vi "START_HERE-Capacitance_Station_Main.vi"() -> ()   [LabVIEW 2020]
uses:
  Global 1.vi
panel:
  out "KeystateHP4275AInitSetup":string
  out "Error OUT : TSL":errorcluster
  out "Voltage Adjusted?":bool
  out "%DiffVoltage":dbl format="%_10g"
  out "VError":dbl format="%_10g"
  out "ReadCurrent":dbl format="%_10g"
  out "ReadVoltage":dbl format="%_10g"
  out "NewBiasVoltage":dbl format="%_10g"
  out "TargetBiasVoltage":dbl format="%_10g"
  out "Iteration Leak Comp":i32
  out "GLOBAL - Test Voltages Array":dbl[](array[numeric])
  out "error out Override":errorcluster
  in  "error in Override":errorcluster
  in  "Specific LCR Frequency ?":bool
  out "ArrayCluster2Arrays":cluster{"DUT (x)":dbl[], "DUT (y)":dbl[]}[](array[cluster])
  out "XY Graph":cluster{"DUT (x)":dbl[], "DUT (y)":dbl[]}[](graph)
  in  "Confirm Min&Max Voltage, Chart Method and Polarity Max Voltage?":bool
  out "Current DUT":i32
  out "Test Finishing : Error Out":errorcluster
  in  "Test Finishing : Error in":errorcluster
  out "error out : Before Test Setup Initialization":errorcluster
  out "error out : After Test Setup Initialization":errorcluster
  out "error out : After Confirm Configuration":errorcluster
  in  "Stop Short Cal":bool
  in  "Stop Open Cal":bool
  out "Frequency":string
  in  "Specific Frequency":T1(ring)=enum."1MHz"
  out "Date (DD/MM/YYYY)":string
  out "Test Type (OUTPUT)":string
  out "Test Fixture (OUTPUT)":string
  in  "Category":T2(ring)
  out "Device Type(OUTPUT)":string
  out "CapRun : error out":errorcluster
  in  "error in 2":errorcluster
  out "Captest?":bool
  out "Test Type":string
  in  "CONFIRM CONFIGURATION?":bool
  out "SHORT Compensation":string
  out "OPEN Compensation":string
  in  "After Cap run":bool
  in  "Generate Report : error in":errorcluster
  out "START PRESSED?":bool
  out "Status : CapRun":bool
  out "Max Test Voltages":dbl
  out "CapTest : Started":bool
  out "CapTest  : current time":timestamp
  out "CapTest CurrDUT : \nElapsed time (minutes)":dbl
  out "DUT   |  Elapsed Time (minutes)":dbl[][](array[numeric])
  in  "CapRun : error in":errorcluster
  out "LowCapMode?":bool
  out "Current Result at \nMax Test Voltages":dbl
  in  "CalOpen : error in":errorcluster
  out "CalShort : current time":timestamp
  out "OpenCal : current time":timestamp
  out "TestSigLevel : current time":timestamp
  in  "Calibration Short : Started":bool
  in  "Open Calibration : Started":bool
  in  "TestSigLevel : Started":bool
  in  "CalShort : error in":errorcluster
  in  "Calibration Short Failed":bool
  in  "Open Calibration Failed":bool
  out "Calibration Short : \nElapsed time (seconds)":dbl
  out "Calibration Open : \nElapsed time (seconds)":dbl
  out "Signal Level : \nElapsed time (seconds)":dbl
  out "Test Voltages (V)":dbl[](array[numeric])
  in  "Polarity for Max Voltage":u16(ring) items=["Positive", "Negative"]
  out "Temporary test data":dbl[][](array[numeric])
  out "error Mult_1":errorcluster
  out "DUT  |  Result":dbl[][](array[numeric])
  in  "DUT":i32=1
  out "Generate Report : error out":errorcluster
  in  "Open Calibration Successful":bool
  in  "Calibration Short Successful":bool
  out "4275A":refnum<visa-resource-name>
  out "3457A":refnum<visa-resource-name>
  out "Keithley 2400":refnum<visa-resource-name>
  in  "Stop":bool
  out "error Mult_0.1":errorcluster
  in  "Min Voltage":dbl
  in  "Start Test":bool
  in  "Max Voltage":dbl
  in  "Chart Voltage Generation Method":u16(ring) items=["Linear", "Crude Semi-Log (Short)", "Crude Semi-Log (Long)", "Bi-directional Crude Semi-Log (Short)", "Bi-directional Crude Semi-Log (Long)", "Manual Fill-In", "Threshold with Increment"]
  in  "Cal Open All Freq":bool
  in  "Cal Short Button":bool
  out "Multiplier":dbl format="%#_3g"
  in  "Device Types":u16(ring) items=["Diode (Rectifier & Zener)", "Transistor", "BRT", "MOSFET", "JFET", "SSOVP", "SIDAC", "Bidirectional Zener", "SCR or TRIAC", "Darlington Transistor", "MicroIntegration", "MOSFET with Gate Resistor", "IGBT", "IGBT with Gate Resistor", "Other"]
  out "Test Level Equal":bool
  in  "Stop Button":bool
  in  "OK Button":bool
  out "Current LCR Voltage":dbl format="%_6g"
  out "Test Level value":dbl
  in  "error in":errorcluster
  in  "Test Signal Level":string(combo)
  in  "Test Comments":string
  in  "Lot Date":timestamp=timestamp(3376684800 s since 1904-01-01) format="%<%x>T"
  in  "Lot Number":string
  in  "Test Fixtures":u16(ring) items=["Diode & Bipolar Capacitance Adapter Box 1, CAP 1, AXK", "Diode & Bipolar Capacitance Adapter Box 1, CAP 2, AXK", "Diode & Bipolar Capacitance Adapter Box 1, CAP 3, Anode - Cathode", "DIODE & BIPOLAR Multi-pin Capacitance fixture"]
  in  "Test System":u16(ring) items=["HP 4275A East Station", "HP 4980A South Station"]
  in  "Part Number":string
  in  "Request Number":string
  out "Report Array Header":string[](array[string])
  in  "Operator":u16(ring) items=["Dan McClurg", "Jason Rall", "Laura Vickers", "Daniel Henscheid", "Dwayne Pierce", "Hannah Morrison", "Charles Reyes", "Fadzly", "Hafiz", "Izwan", "GUEST"]
  # "CAPACITANCE TEST"
  # "FLOW :"
  # "1) Orange"
  # "2) Yellow"
  # "3) Lime"
  # "4) Light Blue"
  # "5) Purple"
  # "6) Red"
  # "RESULT : Capacitance(pF) / RG (Ohm)"
  # "Bias Parameter"
  # "NOTE : Test Signal Level is SEMI-AUTO\n------------------------------------------\nTest Signal Level = Osc Level (V) x Multiplier\n\nRule for Multiplier :\n\nIf Test Signal Level = 1 VRMS,  Multiplier = 1  ;\nElse Multiplier = 0.1\n\nOperator need to adjust Osc Level (V) MANUALLY"
  # "Current Result at Max Voltage before Retest Option"
  # "Verror = Bias - Read\n\nVerror / Bias Voltage\nmust be \nless than 0.001"
  # "Manual Override (OPTIONAL)\n-------------------------------\nSet Specific Frequency\nAFTER choosing TSL"
  # "Bias Current's range : AUTO"
  # "Bias = SourceMeter : K2400"
  # "Read = MultiMeter : HP3457A"
  # "Press 2 Times to Stop"
  # "Error Checking"
  # "LOCATION FOR THESE FILE :\n\ntemp_test_data.csv\ntemp_chart.bmp\n.xls\n\nWILL BE IN C:\\Capacitance_Project"
  # "PRODUCED BY : AFIQAH HASBULLAH ( SBN CZ ENG : 2021)"
  # "Get 4275A Keystate"
  # "This is for Resetting, from \nGlobal Variable"
  # "[] [AN] [BN] [CN] [DN] [FNN]"
  # "Frequency Step\n10 kHz - F11                     1 MHz - F17\n20(30) kHz - F12              2(3) MHz - F18\n40(50) kHz - F13              4(5) MHz - F19\n100 kHz - F14                   10 MHz - F20\n200(300) kHz - F15           *1 - F21\n400(500) kHz - F16           *2 - F22"
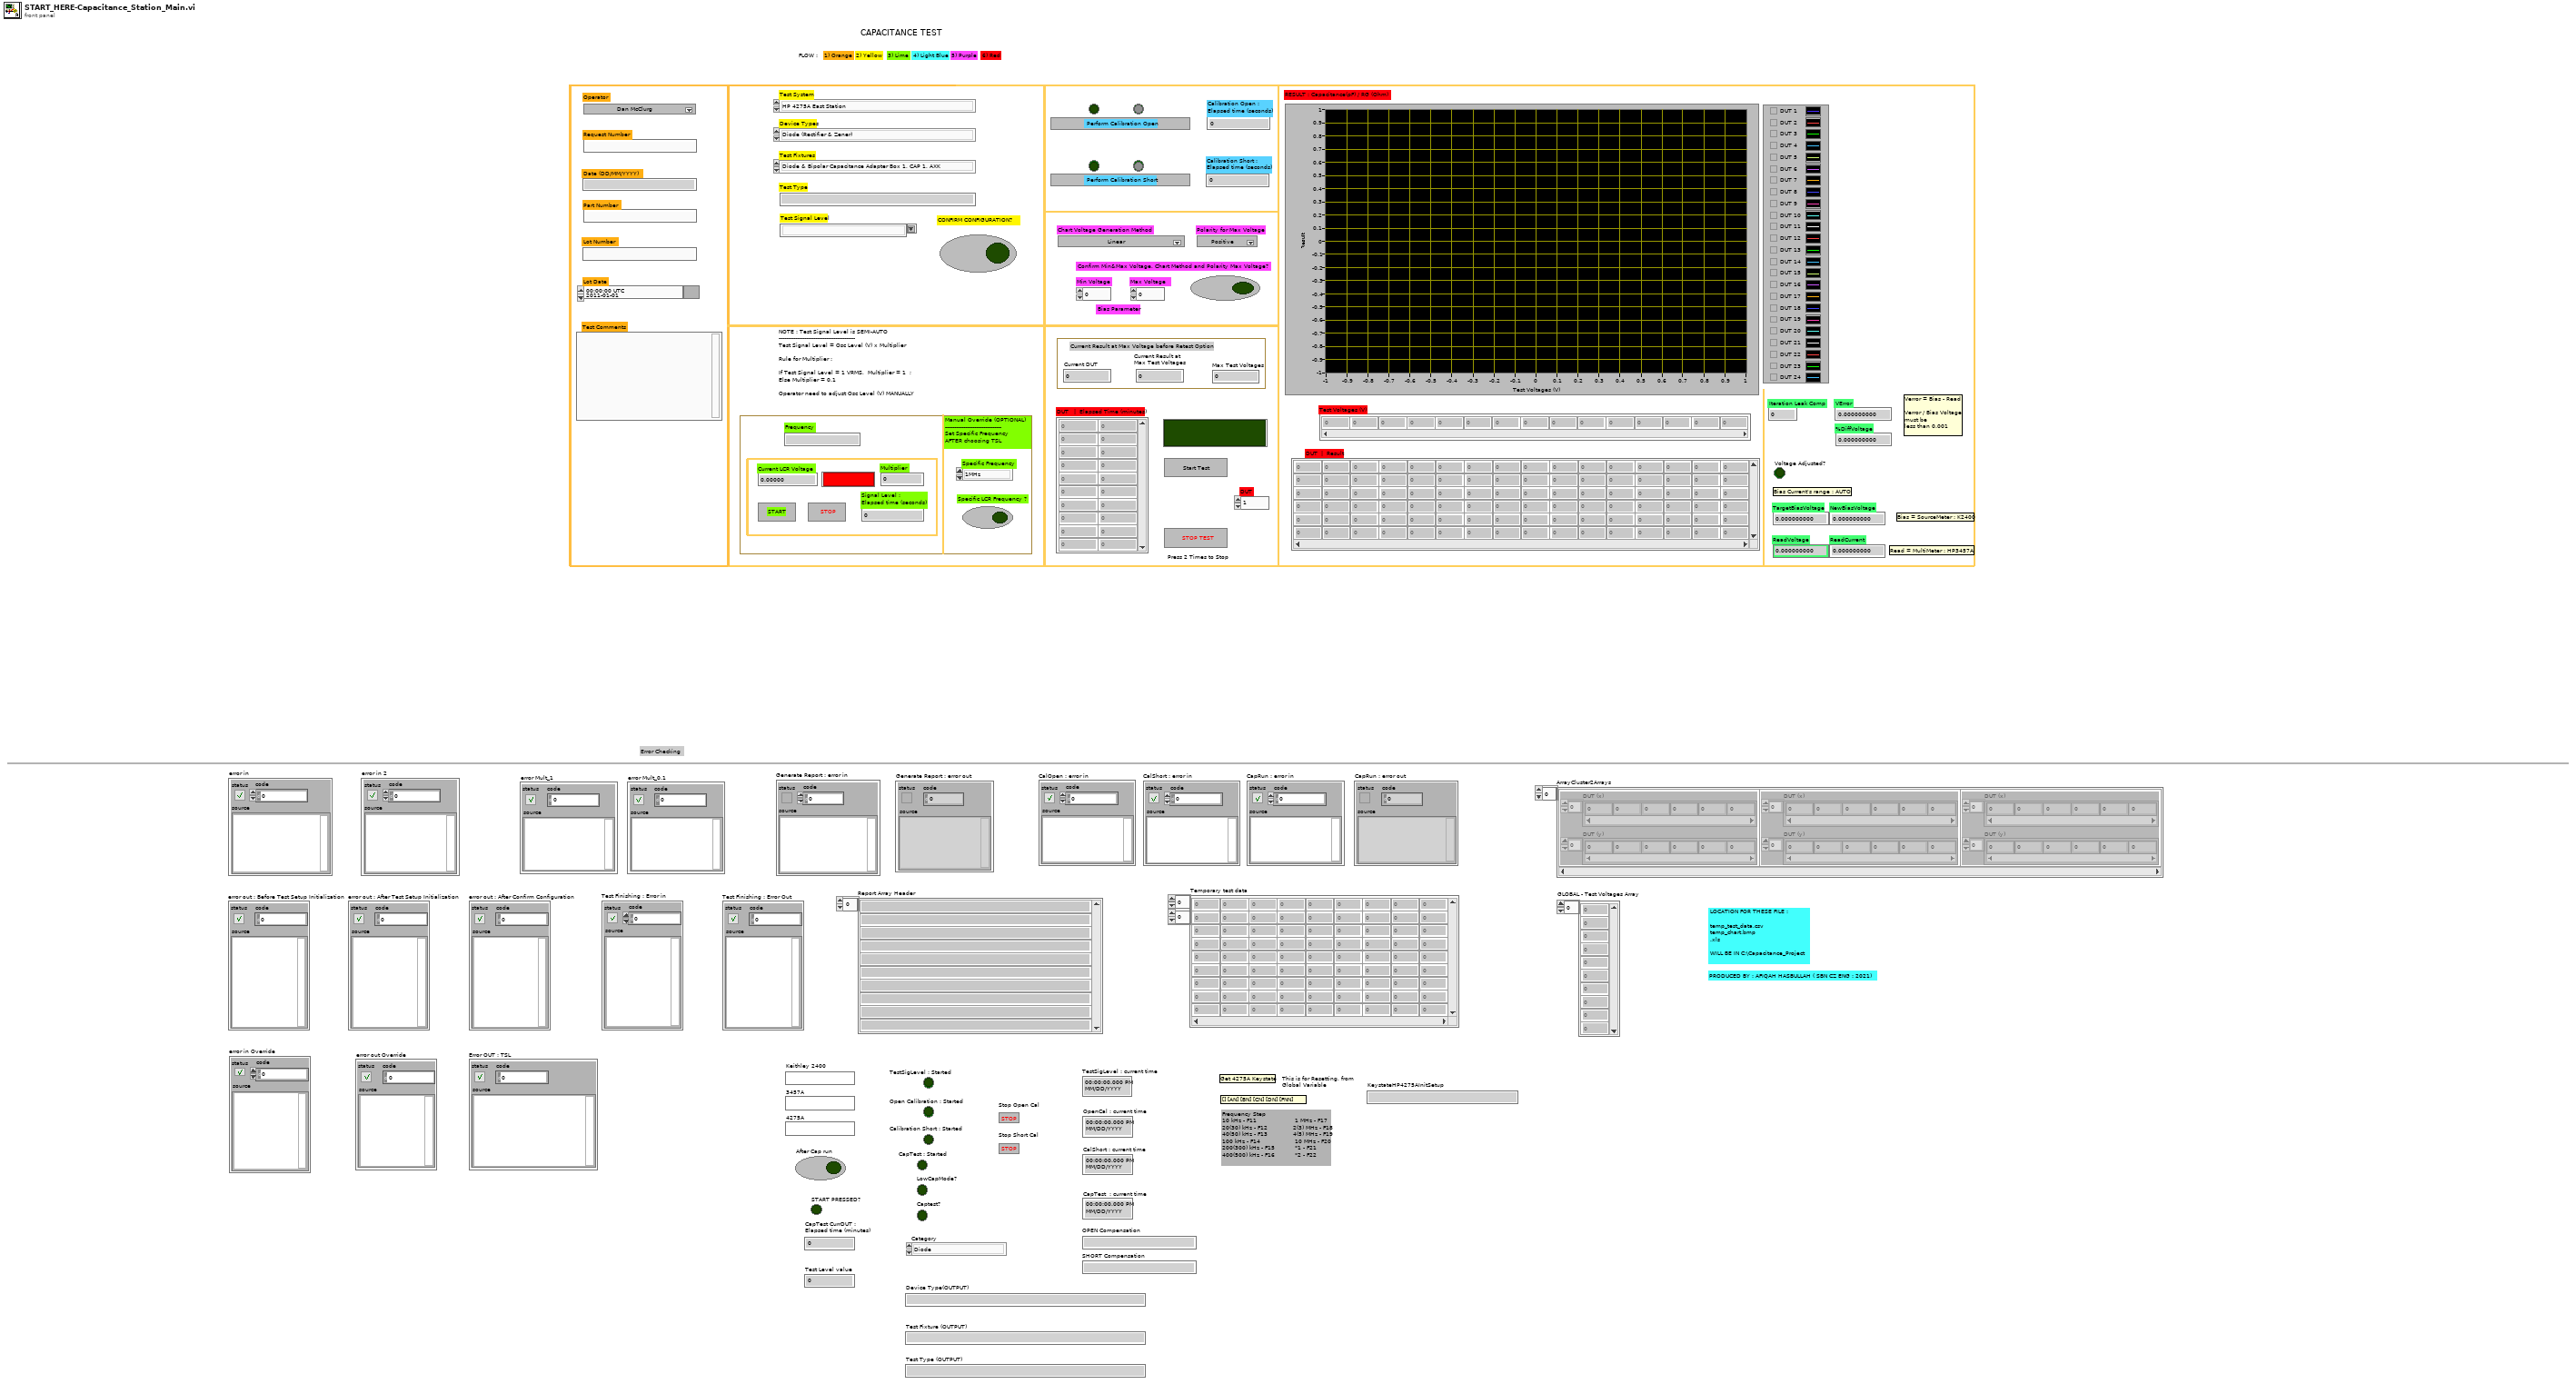
[diagram p1: front panel]
types:
  T1 = enum16{"NULL", "10kHz", "20(30)kHz", "40(50)kHz", "100kHz", "200(300)kHz", "400(500)kHz", "1MHz", "2(3)MHz", "4(5)MHz", "10MHz", "*1", "*2"}
  T2 = enum16{"Diode", "Transistor", "MOSFET", "Thyristor", "IGBT"}
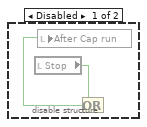
[diagram p3: hidden frame]
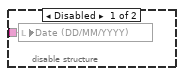
[diagram p4: hidden frame]
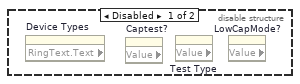
[diagram p7: hidden frame]
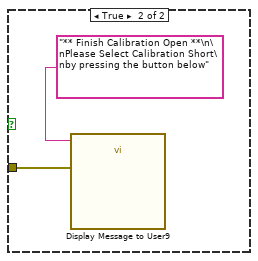
[diagram p15: hidden frame]
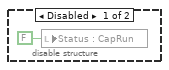
[diagram p19: hidden frame]
diagram:
  # "Manual Override"
  # "Stop Testing, Generate FULL Report"
  # "**********************************STOP **********************************"
  # "Open Calibration, Short Calibration, Start Testing"
  # "**********************************READ & WRITE **********************************"
  # "Initializing Variable"
  # "**********************************START**********************************"
  # "Test Configuration, Report Header, Test Signal Level"
  # "**********************************CONFIGURE**********************************"
  # "LOCAL VARIABLE"
  n1 = disable-structure shown="Enabled" {
    frame Enabled {
      w4 = 0.0
      w6 = 100 ("dimension size")
      w15 = 24 ("dimension size")
      w3 = "" ("Test Type (OUTPUT)")
      w17 = u16 0 items=[""]
      w5 = FALSE
      w13 = 0.0 ("Signal Level : Elapsed time (seconds)")
      w11 = 1 ("Next Part")
      w14 = 0.0 ("element")
      # "Bias Current is always in the range of 10mA"
      # "DUT 24"
      # "DUT 23"
      # "DUT 22"
      # "DUT 21"
      # "DUT 20"
      # "DUT 19"
      # "DUT 18"
      # "DUT 17"
      # "DUT 16"
      # "DUT 15"
      # "DUT 14"
      # "DUT 13"
      # "DUT 12"
      # "DUT 11"
      # "DUT 10"
      # "DUT 9"
      # "DUT 8"
      # "DUT 7"
      # "DUT 6"
      # "DUT 5"
      # "DUT 4"
      # "DUT 3"
      # "DUT 2"
      # "DUT 1"
      # "Array of cluster of Array"
      # "Must have 24 array"
      n2 = Initialize Array(w14, w6, w6) -> (w7:dbl[][])
      n3 = Initialize Array(w14) -> (w24:dbl[])  [unwired: 1 in]
      n4 = Initialize Array(w14, w15, w15) -> (w19:dbl[][])
      n5 = Initialize Array(w14, w15, 2 ("dimension size")) -> (w20:dbl[][])
      n6 = local write "Current DUT"(w11) -> ()
      n7 = local write "DUT"(w11) -> ()
      n8 = local write "Device Types"(w17) -> ()
      n9 = local write "Test Fixtures"(w17) -> ()
      n10 = local write "DUT  |  Result"(w7) -> ()
      n11 = local write "Temporary test data"(w19) -> ()
      n12 = local write "DUT   |  Elapsed Time (minutes)"(w20) -> ()
      n13 = local write "Test Voltages (V)"(w24) -> ()
      n14 = call "Device_GPIB_Addresses.vi"() -> ("HP 4275A Address"=→"4275A":refnum<visa-resource-name>, "HP 3457A Address"=→"3457A":refnum<visa-resource-name>, "Keithley 2400 Address"=→"Keithley 2400":refnum<visa-resource-name>)  [unwired: 9 in]
      n15 = local write "CapTest CurrDUT : \nElapsed time (minutes)"(w13) -> ()
      n16 = local write "Max Test Voltages"(w13) -> ()
      n17 = local write "Current Result at \nMax Test Voltages"(w13) -> ()
      n18 = local write "Signal Level : \nElapsed time (seconds)"(w13) -> ()
      n19 = local write "Calibration Open : \nElapsed time (seconds)"(w13) -> ()
      n20 = local write "Calibration Short : \nElapsed time (seconds)"(w13) -> ()
      n21 = local write "Current LCR Voltage"(w13) -> ()
      n22 = local write "Multiplier"(w13) -> ()
      n23 = local write "XY Graph"(cluster{"DUT (x)":dbl[], "DUT (y)":dbl[]}[] [{"DUT (x)"=[0.0], "DUT (y)"=[0.0]}, {"DUT (x)"=[0.0], "DUT (y)"=[0.0]}, {"DUT (x)"=[0.0], "DUT (y)"=[0.0]}, {"DUT (x)"=[0.0], "DUT (y)"=[0.0]}, {"DUT (x)"=[0.0], "DUT (y)"=[0.0]}, {"DUT (x)"=[0.0], "DUT (y)"=[0.0]}, {"DUT (x)"=[0.0], "DUT (y)"=[0.0]}, {"DUT (x)"=[0.0], "DUT (y)"=[0.0]}, {"DUT (x)"=[0.0], "DUT (y)"=[0.0]}, {"DUT (x)"=[0.0], "DUT (y)"=[0.0]}, {"DUT (x)"=[0.0], "DUT (y)"=[0.0]}, {"DUT (x)"=[0.0], "DUT (y)"=[0.0]}, {"DUT (x)"=[0.0], "DUT (y)"=[0.0]}, {"DUT (x)"=[0.0], "DUT (y)"=[0.0]}, {"DUT (x)"=[0.0], "DUT (y)"=[0.0]}, {"DUT (x)"=[0.0], "DUT (y)"=[0.0]}, {"DUT (x)"=[0.0], "DUT (y)"=[0.0]}, {"DUT (x)"=[0.0], "DUT (y)"=[0.0]}, {"DUT (x)"=[0.0], "DUT (y)"=[0.0]}, {"DUT (x)"=[0.0], "DUT (y)"=[0.0]}, {"DUT (x)"=[0.0], "DUT (y)"=[0.0]}, {"DUT (x)"=[0.0], "DUT (y)"=[0.0]}, {"DUT (x)"=[0.0], "DUT (y)"=[0.0]}, {"DUT (x)"=[0.0], "DUT (y)"=[0.0]}] ("Array of DUT Cluster")) -> ()
      n24 = disable-structure shown="Enabled" {
        frame Enabled {
          w30 = "" ("KeystateHP4275AInitSetup")
          w29 = 0 ("Array Size")
          # "Global Variable Initialization"
          n25 = Initialize Array(0.0 ("element")) -> (w33:dbl[])  [unwired: 1 in]
          n26 = global write "Global 1.vi" "KeystateHP4275AInitSetup"(w30) -> ()
          n27 = global write "Global 1.vi" "Device Type-GB"(w30) -> ()
          n28 = global write "Global 1.vi" "Test Type-GB"(w30) -> ()
          n29 = global write "Global 1.vi" "Test Comment-GB"(w30) -> ()
          n30 = global write "Global 1.vi" "Array Size"(w29) -> ()
          n31 = global write "Global 1.vi" "Iteration Leak Comp"(w29) -> ()
          n32 = global write "Global 1.vi" "DUT"(w29) -> ()
          n33 = global write "Global 1.vi" "Result - Test Voltages Array"(w33) -> ()
          n34 = global write "Global 1.vi" "~~ FINISH ~~"(FALSE ("~~ FINISH ~~")) -> ()
          n35 = global write "Global 1.vi" "error out"(errorcluster {"status"=FALSE, "code"=0, "source"=""} ("error out")) -> ()
        }
        frame Disabled {
        }
      }
      n36 = local write "%DiffVoltage"(w4) -> ()
      n37 = local write "VError"(w4) -> ()
      n38 = local write "ReadCurrent"(w4) -> ()
      n39 = local write "ReadVoltage"(w4) -> ()
      n40 = local write "NewBiasVoltage"(w4) -> ()
      n41 = local write "TargetBiasVoltage"(w4) -> ()
      n42 = global write "Global 1.vi" "%DiffVoltage"(w4) -> ()
      n43 = global write "Global 1.vi" "NewBiasVoltage"(w4) -> ()
      n44 = global write "Global 1.vi" "TargetBiasVoltage"(w4) -> ()
      n45 = global write "Global 1.vi" "ReadVoltage"(w4) -> ()
      n46 = global write "Global 1.vi" "ReadCurrent"(w4) -> ()
      n47 = global write "Global 1.vi" "VError"(w4) -> ()
      n48 = local write "KeystateHP4275AInitSetup"(w3) -> ()
      n49 = local write "Device Type(OUTPUT)"(w3) -> ()
      n50 = disable-structure shown="Enabled" {
        disable-tunnel: w3 -> [w28 _]
        frame Disabled {
          n51 = local write "Date (DD/MM/YYYY)"(w28) -> ()
        }
        frame Enabled {
        }
      }
      n52 = local write "Test Type (OUTPUT)"(w3) -> ()
      n53 = local write "Test Fixture (OUTPUT)"(w3) -> ()
      n54 = local write "Frequency"(w3) -> ()
      n55 = local write "Test Type"(w3) -> ()
      n56 = local write "OPEN Compensation"(w3) -> ()
      n57 = local write "SHORT Compensation"(w3) -> ()
      n58 = local write "Report Array Header"(string[] ["", "", "", "", "", "", "", "", "", "", "", "", "", "", ""] ("Report Array Header")) -> ()
      n59 = local write "Specific LCR Frequency ?"(w5) -> ()
      n60 = local write "Voltage Adjusted?"(w5) -> ()
      n61 = global write "Global 1.vi" "Voltage Adjusted?"(w5) -> ()
      n62 = local write "Stop Open Cal"(w5) -> ()
      n63 = local write "Stop Short Cal"(w5) -> ()
      n64 = local write "Test Level Equal"(w5) -> ()
      n65 = local write "Confirm Min&Max Voltage, Chart Method and Polarity Max Voltage?"(w5) -> ()
      n66 = local write "OK Button"(w5) -> ()
      n67 = local write "Stop Button"(w5) -> ()
      n68 = local write "After Cap run"(w5) -> ()
      n69 = local write "CapTest : Started"(w5) -> ()
      n70 = local write "LowCapMode?"(TRUE ("LowCapMode?")) -> ()
      n71 = local write "CONFIRM CONFIGURATION?"(w5) -> ()
      n72 = local write "Captest?"(TRUE ("Captest?")) -> ()
      n73 = local write "Calibration Short Successful"(w5) -> ()
      n74 = local write "Status : CapRun"(w5) -> ()
      n75 = local write "Calibration Short Failed"(w5) -> ()
      n76 = local write "Open Calibration Failed"(w5) -> ()
      n77 = local write "Cal Short Button"(w5) -> ()
      n78 = local write "Cal Open All Freq"(w5) -> ()
      n79 = local write "Open Calibration Successful"(w5) -> ()
      n80 = local write "Calibration Short : Started"(w5) -> ()
      n81 = local write "Open Calibration : Started"(w5) -> ()
      n82 = local write "TestSigLevel : Started"(w5) -> ()
      n83 = local write "Start Test"(w5) -> ()
      n84 = local write "Stop"(w5) -> ()
      n85 = local write "Specific LCR Frequency ?"(FALSE ("Specific LCR Frequency ?")) -> ()
      n86 = local write "CapTest  : current time"(timestamp(0 s since 1904-01-01) ("CapTest  : current time")) -> ()
      n87 = local write "TestSigLevel : current time"(timestamp(0 s since 1904-01-01) ("TestSigLevel : current time")) -> ()
      n88 = local write "OpenCal : current time"(timestamp(0 s since 1904-01-01) ("OpenCal : current time")) -> ()
      n89 = local write "CalShort : current time"(timestamp(0 s since 1904-01-01) ("CalShort : current time")) -> ()
      n90 = local write "Specific Frequency"(T1."1MHz" ("Specific Frequency")) -> ()
    }
    frame Disabled {
    }
  }
  n91 = disable-structure shown="Enabled" {
    frame Enabled {
      # "CALL ConfigGPIB\nCALL ConfigK2400\nCALL ResetHP3457\nCALL ConfigHP3457Norm"
      # "Captest?"
      # "Set Header"
      # "Test Type (OUTPUT)"
      # "Test Fixture (OUTPUT)"
      n92 = flat-sequence {
        tunnel: [w94] -> w54
        tunnel: [w93] -> w53
        tunnel: [w92] -> w52
        tunnel: [w91] -> w48
        tunnel: [w90] -> w45
        tunnel: [w89] -> w43
        tunnel: [w88] -> w39
        tunnel: [w101] -> w56
        tunnel: [w108] -> w55
        tunnel: w54 -> [w108]
        tunnel: [w107] -> w49
        tunnel: w48 -> [w107]
        tunnel: [w106] -> w46
        tunnel: w45 -> [w106]
        tunnel: [w105] -> w44
        tunnel: w43 -> [w105]
        tunnel: w39 -> [w102]
        tunnel: w56 -> [w118]
        tunnel: w55 -> [w117]
        tunnel: [w115] -> w50
        tunnel: w49 -> [w113]
        tunnel: [w113] -> w47
        tunnel: w46 -> [w112]
        tunnel: w44 -> [w110]
        frame #0 {
          n93 = control-ref of="Test Signal Level"() -> (w98:refnum<vi>)
          n94 = control-ref of="Device Types"() -> (w94:refnum<vi>)
          n95 = control-ref of="Test Fixtures"() -> (w97:refnum<vi>)
          n96 = control-ref of="Test Type"() -> (w89:refnum<vi>)
          n97 = control-ref of="CONFIRM CONFIGURATION?"() -> (w100:refnum<vi>)
          n98 = control-ref of="Category"() -> (w96:refnum<vi>)
          n99 = control-ref of="Captest?"() -> (w91:refnum<vi>)
          n100 = control-ref of="Device Type(OUTPUT)"() -> (w99:refnum<vi>)
          n101 = control-ref of="Test Fixture (OUTPUT)"() -> (w92:refnum<vi>)
          n102 = control-ref of="Test Type (OUTPUT)"() -> (w93:refnum<vi>)
          n103 = control-ref of="LowCapMode?"() -> (w90:refnum<vi>)
          n104 = call "Ref_Num_Test_Conf.vi"("Device Types"=w94, "Test Fixtures"=w97, "Test Signal Level"=w98, "Device Type (OUTPUT)"=w99, "Test Types"=w89, "Test Fixture (OUTPUT)"=w92, "Confirm Configuration"=w100, "Test Type (OUTPUT)"=w93, "error in"="error in 2", "Category"=w96, "LowCapMode?"=w90, "CAPACITANCE TEST?"=w91) -> ("error out"=w88:errorcluster)  [unwired: 3 in]
        }
        frame #1 {
          # "Wait until \nConfiguration Confirmed"
          n105 = call "Message_dialog.vi"("error in (no error)"=w102, "set delay"=2.0, "String"="Test Configuration will be Set Up\nPlease Wait...\n\n") -> ("error out"=w101:errorcluster)  [unwired: 8 in]
        }
        frame #2 {
          # "Test Type"
          # "LowCapMode?"
          # "Captest?"
          # "Device Types"
          # "Test Mode\nTrue : Cap"
          # "AUTO RANGING"
          # "RESOLUTION SETUP"
          # "Mode Setup"
          # "Default - C"
          # "FET Test Config"
          n106 = property class="Bool (strict)"(reference=w112) -> ("Value"=w111:bool)  [unwired: 1 in, 2 out]
          n107 = property class="Bool (strict)"(reference=w113) -> ("Value"=w114:bool)  [unwired: 1 in, 2 out]
          n108 = property class="Ring (strict)"(reference=w117) -> ("RingText.Text"=w116:string)  [unwired: 1 in, 2 out]
          n109 = global write "Global 1.vi" "Device Type-GB"(w116) -> ()
          n110 = property class="Str"(reference=w110) -> ("Value"=w109:string)  [unwired: 1 in, 2 out]
          n111 = global write "Global 1.vi" "Test Type-GB"(w109) -> ()
          n112 = call "FET_Test_Config_4275A.vi"("LowCapMode?"=w111, "error in"=w118, "Test Mode"=w114, "Device Type"=w116, "FET Test Configuration"=w109) -> ("error out"=w115:errorcluster)  [unwired: 6 in]
        }
      }
      n113 = disable-structure shown="Enabled" {
        disable-tunnel: [w122 _] -> w42
        disable-tunnel: "error in" -> [w121 _]
        frame Enabled {
          # "Test Setup Initialization"
          n114 = while {
            shift-right: [w128] -> w120
            shift-left: w121 -> [w129]
            stop <- w127 stop-if-true
            n115 = call <vilib>:"Beep.vi"("use system alert? (T)"=FALSE, "duration (msec)"=u32 3000, "frequency (Hz)"=u32 1000) -> ()  [unwired: 9 in]
            n116 = call "Display Message to User8"("error in (no error)"=w129) -> ("error out"=w128:errorcluster, "OK"=w127:bool)  [unwired: 9 in]
            n117 = Wait (ms)(milliseconds to wait=u32 200) -> ()  [unwired: 1 out]
          }
          "error out : Before Test Setup Initialization" <- w120
          n118 = call "Test_Setup_Initialization.vi"("HP 3457A Error In"=w120) -> ("HP 3457A Error Out"=w119:errorcluster)  [unwired: 10 in]
          "error out : After Test Setup Initialization" <- w119
          n119 = while {
            shift-right: [w132] -> w122
            shift-left: w119 -> [w133]
            stop <- w131 stop-if-true
            n120 = call "Display Message to User7"("error in (no error)"=w133) -> ("error out"=w132:errorcluster, "OK"=w131:bool)  [unwired: 9 in]
            n121 = Wait (ms)(milliseconds to wait=u32 200) -> ()  [unwired: 1 out]
          }
        }
        frame Disabled {
        }
      }
      n122 = disable-structure shown="Enabled" {
        frame Disabled {
          n123 = property on="Device Types" class="Ring (strict)" props=["RingText", "Text"]() -> ()  [unwired: 2 in, 3 out]
          n124 = property on="Captest?" class="Bool (strict)" props=["Value"]() -> ()  [unwired: 2 in, 3 out]
          n125 = property on="Test Type" class="Str" props=["Value"]() -> ()  [unwired: 2 in, 3 out]
          n126 = property on="LowCapMode?" class="Bool (strict)" props=["Value"]() -> ()  [unwired: 2 in, 3 out]
        }
        frame Enabled {
        }
      }
      n127 = global read "Global 1.vi" "Test Comment-GB"() -> (w51:string)
      n128 = control-ref of="Current LCR Voltage"() -> (w83:refnum<vi>)
      n129 = control-ref of="Test Level value"() -> (w84:refnum<vi>)
      n130 = control-ref of="Frequency"() -> (w57:refnum<vi>)
      n131 = control-ref of="OPEN Compensation"() -> (w81:refnum<vi>)
      n132 = control-ref of="SHORT Compensation"() -> (w82:refnum<vi>)
      n133 = control-ref of="Report Array Header"() -> (w87:refnum<vi>)
      n134 = control-ref of="Operator"() -> (w86:refnum<vi>)
      n135 = control-ref of="Request Number"() -> (w85:refnum<vi>)
      n136 = Merge Errors(w50, w42) -> (w60:errorcluster)
      n137 = control-ref of="Specific LCR Frequency ?"() -> (w36:refnum<vi>)
      n138 = control-ref of="Specific Frequency"() -> (w35:refnum<vi>)
      n139 = while {
        shift-right: [w136] -> w59
        shift-left: w60 -> [w137]
        stop <- w135 stop-if-true
        n140 = call "Display Message to User2"("error in (no error)"=w137) -> ("error out"=w136:errorcluster, "OK"=w135:bool)  [unwired: 9 in]
        n141 = Wait (ms)(milliseconds to wait=u32 200) -> ()  [unwired: 1 out]
      }
      n142 = control-ref of="Stop"() -> (w41:refnum<vi>)
      n143 = control-ref of="Date (DD/MM/YYYY)"() -> (w78:refnum<vi>)
      n144 = control-ref of="Lot Date"() -> (w77:refnum<vi>)
      n145 = call "Ref_Num_OverrideSpec.vi"("error in"="error in Override", "Specific Frequency"=w35, "Set LCR Frequency"=w36) -> ("error out"=→"error out Override":errorcluster)  [unwired: 8 in]
      n146 = control-ref of="Open Calibration : Started"() -> (w79:refnum<vi>)
      n147 = control-ref of="Calibration Short : Started"() -> (w80:refnum<vi>)
      n148 = control-ref of="Part Number"() -> (w76:refnum<vi>)
      n149 = control-ref of="Test Comments"() -> (w73:refnum<vi>)
      n150 = control-ref of="Lot Number"() -> (w74:refnum<vi>)
      n151 = control-ref of="Test System"() -> (w75:refnum<vi>)
      n152 = call "Ref_Num_Set_Header.vi"("Report Array Header"=w87, "Test Fixture (OUTPUT)"=w52, "Frequency"=w57, "Test Type (OUTPUT)"=w53, "AddTestComment"=w51, "Test Level value"=w84, "Current LCR Voltage"=w83, "Operator"=w86, "SHORT Compensation"=w82, "Request Number"=w85, "OPEN Compensation"=w81, "Date (DD/MM/YYYY)"=w78, "Calibration Short : Started"=w80, "Captest?"=w47, "Open Calibration : Started"=w79, "Lot Date"=w77, "Part Number"=w76, "Test System"=w75, "Lot Number"=w74, "Test Comments"=w73, "Stop"=w41) -> ()  [unwired: 7 in]
      n153 = control-ref of="Test Signal Level"() -> (w64:refnum<vi>)
      n154 = control-ref of="TestSigLevel : Started"() -> (w63:refnum<vi>)
      n155 = control-ref of="Multiplier"() -> (w65:refnum<vi>)
      n156 = control-ref of="OK Button"() -> (w62:refnum<vi>)
      n157 = control-ref of="Stop Button"() -> (w61:refnum<vi>)
      n158 = control-ref of="Test Level Equal"() -> (w66:refnum<vi>)
      n159 = control-ref of="Test Level value"() -> (w67:refnum<vi>)
      n160 = control-ref of="Current LCR Voltage"() -> (w68:refnum<vi>)
      n161 = control-ref of="TestSigLevel : current time"() -> (w69:refnum<vi>)
      n162 = control-ref of="Signal Level : \nElapsed time (seconds)"() -> (w70:refnum<vi>)
      n163 = call "Ref_Num_Set_VRMS.vi"("Multiplier"=w65, "Test Level Equal"=w66, "Test Level value"=w67, "Current LCR Voltage"=w68, "TestSigLevel : current time"=w69, "Test Signal Level"=w64, "Signal Level : Elapsed time (seconds)"=w70, "error IN"=w59, "TestSigLevel : Started"=w63, "OK Button"=w62, "Stop Button"=w61) -> ("Error OUT"=→"Error OUT : TSL":errorcluster, "error Mult_0.1"=→"error Mult_0.1":errorcluster, "error Mult_1"=→"error Mult_1":errorcluster)  [unwired: 2 in]
      "error out : After Confirm Configuration" <- w50
    }
    frame Disabled {
    }
  }
  n164 = disable-structure shown="Enabled" {
    frame Enabled {
      # "Capacitance Test"
      # "Needs to be looked at and verified."
      n165 = control-ref of="Stop"() -> (w146:refnum<vi>)
      n166 = control-ref of="After Cap run"() -> (w147:refnum<vi>)
      n167 = control-ref of="Start Test"() -> (w145:refnum<vi>)
      n168 = control-ref of="CapTest CurrDUT : \nElapsed time (minutes)"() -> (w142:refnum<vi>)
      n169 = control-ref of="Current DUT"() -> (w138:refnum<vi>)
      n170 = control-ref of="DUT"() -> (w143:refnum<vi>)
      n171 = control-ref of="DUT   |  Elapsed Time (minutes)"() -> (w144:refnum<vi>)
      n172 = while {
        tunnel: w147 -> [w189]
        tunnel: w146 -> [w188]
        tunnel: w145 -> [w184]
        tunnel: w144 -> [w187]
        tunnel: w143 -> [w186]
        tunnel: w142 -> [w185]
        tunnel: w138 -> [w170]
        stop <- w174 stop-if-true
        n173 = global read "Global 1.vi" "Result - Test Voltages Array"() -> (→"GLOBAL - Test Voltages Array":dbl[])
        n174 = global read "Global 1.vi" "ArrayCluster2Arrays"() -> (→"ArrayCluster2Arrays":cluster{"DUT (x)":dbl[], "DUT (y)":dbl[]}[])
        n175 = global read "Global 1.vi" "Iteration Leak Comp"() -> (→"Iteration Leak Comp":i32)
        n176 = property class="Bool (strict)"(reference=w188) -> ("Value"=w174:bool)  [unwired: 1 in, 2 out]
        n177 = Wait (ms)(milliseconds to wait=u32 200) -> ()  [unwired: 1 out]
        n178 = global read "Global 1.vi" "%DiffVoltage"() -> (w175:dbl)
        n179 = global read "Global 1.vi" "NewBiasVoltage"() -> (w179:dbl)
        n180 = property class="Bool (strict)"(reference=w189, "Value"=w174) -> ()  [unwired: 1 in, 2 out]
        n181 = global read "Global 1.vi" "TargetBiasVoltage"() -> (w180:dbl)
        n182 = global read "Global 1.vi" "ReadVoltage"() -> (w178:dbl)
        n183 = global read "Global 1.vi" "ReadCurrent"() -> (w177:dbl)
        n184 = global read "Global 1.vi" "VError"() -> (w176:dbl)
        n185 = property class="Bool (strict)"(reference=w184) -> ("Value"=w193:bool)  [unwired: 1 in, 2 out]
        n186 = local write "ReadCurrent"(w177) -> ()
        n187 = local write "VError"(w176) -> ()
        n188 = local write "%DiffVoltage"(w175) -> ()
        n189 = local write "NewBiasVoltage"(w179) -> ()
        n190 = local write "ReadVoltage"(w178) -> ()
        n191 = local write "TargetBiasVoltage"(w180) -> ()
        n192 = Equal?(x=w193, y=TRUE) -> (x = y?=w191:bool)
        "START PRESSED?" <- w191
        n193 = global read "Global 1.vi" "KeystateHP4275AInitSetup"() -> (w172:string)
        n194 = global read "Global 1.vi" "Voltage Adjusted?"() -> (w173:bool)
        n195 = case shown="True" w191 {
          tunnel: w187 -> [_ w198]
          tunnel: w186 -> [_ w197]
          tunnel: w185 -> [_ w196]
          tunnel: w170 -> [_ w194]
          frame False {
          }
          frame True {
            n196 = property class="DigNum (strict)"(reference=w197) -> ("Value"=w195:i32)  [unwired: 1 in, 2 out]
            n197 = property class="DigNum (strict)"(reference=w194, "Value"=w195) -> ()  [unwired: 1 in, 2 out]
            n198 = property class="DigNum (strict)"(reference=w196) -> ("Value"=w205:dbl)  [unwired: 1 in, 2 out]
            n199 = Subtract(x=w195, y=1) -> (x-y=w201:i32)
            n200 = property class="Arr (strict)"(reference=w198) -> ("Value"=w203:dbl[][])  [unwired: 1 in, 2 out]
            n201 = To Double Precision Float(number=w195) -> (double precision float=w200:dbl)
            n202 = Build Array(w200, w205) -> (w202:dbl[])
            n203 = Replace Array Subset(array=w203, new element=w202, index (row)=w201) -> (w204:dbl[][])  [unwired: 1 in]
            n204 = property class="Arr (strict)"(reference=w198, "Value"=w204) -> ()  [unwired: 1 in, 2 out]
          }
        }
        n205 = local read "DUT"() -> (w171:i32)
        n206 = local write "Voltage Adjusted?"(w173) -> ()
        n207 = local write "KeystateHP4275AInitSetup"(w172) -> ()
        n208 = global write "Global 1.vi" "DUT"(w171) -> ()
      }
      n209 = control-ref of="XY Graph"() -> (w148:refnum<vi>)
      n210 = control-ref of="Start Test"() -> (w156:refnum<vi>)
      n211 = control-ref of="LowCapMode?"() -> (w165:refnum<vi>)
      n212 = control-ref of="Confirm Min&Max Voltage, Chart Method and Polarity Max Voltage?"() -> (w152:refnum<vi>)
      n213 = control-ref of="DUT  |  Result"() -> (w164:refnum<vi>)
      n214 = control-ref of="Test Voltages (V)"() -> (w162:refnum<vi>)
      n215 = control-ref of="Max Test Voltages"() -> (w154:refnum<vi>)
      n216 = control-ref of="Stop"() -> (w166:refnum<vi>)
      n217 = control-ref of="Polarity for Max Voltage"() -> (w158:refnum<vi>)
      n218 = control-ref of="Current Result at \nMax Test Voltages"() -> (w159:refnum<vi>)
      n219 = control-ref of="Chart Voltage Generation Method"() -> (w157:refnum<vi>)
      n220 = control-ref of="Status : CapRun"() -> (w155:refnum<vi>)
      n221 = control-ref of="Min Voltage"() -> (w161:refnum<vi>)
      n222 = control-ref of="Max Voltage"() -> (w160:refnum<vi>)
      n223 = control-ref of="DUT"() -> (w153:refnum<vi>)
      n224 = control-ref of="Captest?"() -> (w163:refnum<vi>)
      n225 = call "Ref_Num_Generate_Report_NEW.vi"("LowCapMode?"=w165, "Test Part"=w156, "Test Voltages(V)"=w154, "T.V. True"=w152, "Stop"=w166, "error in (no error)"="CapRun : error in", "Array"=w164, "Chart Voltage Generation Method"=w157, "XY Graph NEW"=w148, "CapTest?"=w163, "Polarity for Max Voltage"=w158, "Test Voltages Chosen"=w162, "Capacitance(pF)"=w159, "Min Voltage"=w161, "Max Voltage"=w160, "Status : Running"=w155, "Next Part"=w153) -> ("error out"=→"CapRun : error out":errorcluster)  [unwired: 2 in]
      n226 = control-ref of="Stop"() -> (w140:refnum<vi>)
      n227 = control-ref of="Start Test"() -> (w141:refnum<vi>)
      n228 = control-ref of="CapTest : Started"() -> (w150:refnum<vi>)
      n229 = property class="Bool (strict)"(reference=w141) -> ("Value"=w139:bool)  [unwired: 1 in, 2 out]
      n230 = control-ref of="CapTest CurrDUT : \nElapsed time (minutes)"() -> (w149:refnum<vi>)
      n231 = control-ref of="CapTest  : current time"() -> (w151:refnum<vi>)
      n232 = call "Ref_Num_Stopwatch_CapTest.vi"("Elapsed time (seconds)"=w149, "start time"=w151, "stop"=w140, "OK Button"=w141, "Started"=w150) -> ()  [unwired: 7 in]
      n233 = case shown="True" w139 {
        frame False {
        }
        frame True {
          n234 = Get Date/Time In Seconds() -> (seconds since 1Jan1904=→"CapTest  : current time":timestamp)
        }
      }
    }
    frame Disabled {
    }
  }
  n235 = disable-structure shown="Enabled" {
    frame Enabled {
      # "Calibration Open"
      n236 = control-ref of="Stop Open Cal"() -> (w210:refnum<vi>)
      n237 = control-ref of="LowCapMode?"() -> (w213:refnum<vi>)
      n238 = control-ref of="Cal Open All Freq"() -> (w214:refnum<vi>)
      n239 = control-ref of="Open Calibration : Started"() -> (w217:refnum<vi>)
      n240 = control-ref of="Open Calibration Successful"() -> (w212:refnum<vi>)
      n241 = property class="Bool (strict)"(reference=w214) -> ("Value"=w218:bool)  [unwired: 1 in, 2 out]
      n242 = control-ref of="Open Calibration Failed"() -> (w220:refnum<vi>)
      n243 = call "Ref_Num_Calibrate_Open.vi"("Test Failed"=w220, "Open Calibration Successful"=w212, "error in"="CalOpen : error in", "Stop Test"=w210, "LowCapMode?"=w213, "Calibration Test"=w214) -> ("error out"=w211:errorcluster)  [unwired: 5 in]
      n244 = case shown="True" w218 {
        frame False {
        }
        frame True {
          n245 = Get Date/Time In Seconds() -> (seconds since 1Jan1904=→"OpenCal : current time":timestamp)
        }
      }
      n246 = control-ref of="Test Type"() -> (w209:refnum<vi>)
      n247 = control-ref of="OpenCal : current time"() -> (w215:refnum<vi>)
      n248 = control-ref of="Calibration Open : \nElapsed time (seconds)"() -> (w216:refnum<vi>)
      n249 = call "Ref_Num_Stopwatch_Op.vi"("Elapsed time (seconds)"=w216, "start time"=w215, "Started"=w217, "OK Button"=w214, "stop"=w212) -> ()  [unwired: 1 in]
      n250 = property class="Str"(reference=w209) -> ("Value"=w208:string)  [unwired: 1 in, 2 out]
      n251 = Equal?(x=w208, y="RG") -> (x = y?=w206:bool)
      n252 = case shown="False" w206 {
        tunnel: w211 -> [w221 w223]
        frame False {
          n253 = call "Display Message to User3"("error in (no error)"=w221, "Message"="** Finish Calibration Open **\n\nCan Continue with Chart Method,\nBias Parameter & Run Full Test in the \nRow Below" ("message")) -> ()  [unwired: 8 in, 2 out]
        }
        frame True {
          n254 = call "Display Message to User9"("error in (no error)"=w223, "Message"="** Finish Calibration Open **\n\nPlease Select Calibration Short\nby pressing the button below" ("message")) -> ()  [unwired: 8 in, 2 out]
        }
      }
    }
    frame Disabled {
    }
  }
  n255 = disable-structure shown="Enabled" {
    frame Enabled {
      # "Calibration Short/Rg"
      n256 = control-ref of="Stop Short Cal"() -> (w226:refnum<vi>)
      n257 = control-ref of="Cal Short Button"() -> (w229:refnum<vi>)
      n258 = control-ref of="Calibration Short : Started"() -> (w231:refnum<vi>)
      n259 = control-ref of="Calibration Short Successful"() -> (w227:refnum<vi>)
      n260 = control-ref of="LowCapMode?"() -> (w228:refnum<vi>)
      n261 = property class="Bool (strict)"(reference=w229) -> ("Value"=w230:bool)  [unwired: 1 in, 2 out]
      n262 = control-ref of="Calibration Short Failed"() -> (w235:refnum<vi>)
      n263 = call "Ref_Num_Calibrate_Short.vi"("Test Failed"=w235, "Calibration Short Successful"=w227, "LowCapMode?"=w228, "error in"="CalShort : error in", "Stop Test"=w226, "Calibration Test"=w229) -> ("error out"=w237:errorcluster)  [unwired: 5 in]
      n264 = control-ref of="Calibration Short : \nElapsed time (seconds)"() -> (w233:refnum<vi>)
      n265 = control-ref of="CalShort : current time"() -> (w232:refnum<vi>)
      n266 = call "Ref_Num_Stopwatch_Sh.vi"("Elapsed time (seconds)"=w233, "start time"=w232, "Started"=w231, "OK Button"=w229, "stop"=w227) -> ()  [unwired: 1 in]
      n267 = case shown="True" w230 {
        frame False {
        }
        frame True {
          n268 = Get Date/Time In Seconds() -> (seconds since 1Jan1904=→"CalShort : current time":timestamp)
        }
      }
      n269 = call "Display Message to User4"("error in (no error)"=w237, "Message"="** Finish Calibration Short **\n\nCan Continue with Chart Method,\nBias Parameter & Run Full Test in the \nRow Below" ("message")) -> ()  [unwired: 8 in, 2 out]
    }
    frame Disabled {
    }
  }
  n270 = disable-structure shown="Disabled" {
    frame Disabled {
      n271 = while {
        stop <- w239 stop-if-true
        n272 = control-ref of="Stop"() -> (w241:refnum<vi>)
        n273 = property class="Bool (strict)"(reference=w241) -> ("Value"=w239:bool)  [unwired: 1 in, 2 out]
        n274 = control-ref of="After Cap run"() -> (w240:refnum<vi>)
        n275 = property class="Bool (strict)"(reference=w240, "Value"=w239) -> ()  [unwired: 1 in, 2 out]
      }
    }
    frame Enabled {
    }
  }
  n276 = while {
    stop <- w242 stop-if-true
    n277 = control-ref of="After Cap run"() -> (w247:refnum<vi>)
    n278 = property class="Bool (strict)"(reference=w247) -> ("Value"=w243:bool)  [unwired: 1 in, 2 out]
    n279 = control-ref of="Stop"() -> (w245:refnum<vi>)
    n280 = property class="Bool (strict)"(reference=w245) -> ("Value"=w244:bool)  [unwired: 1 in, 2 out]
    n281 = Wait (ms)(milliseconds to wait=u32 200) -> ()  [unwired: 1 out]
    n282 = Or(x=w244, y=w243) -> (x .or. y?=w242:bool)
    n283 = case shown="True" w242 {
      frame False {
      }
      frame True {
        # "Set_K2400_Zero"
        # "Config_3457_Norm"
        # "Test Setup Finishing"
        # "Turn Off Output K2400"
        # "DONE : \n-> Transfer data from temporary csv to xls\n->Use hardcodded VBA Macro, must enabled Macro in Excel Trust Centre\n-> Perfecting the header format as in Panda"
        # "Report Generation"
        # "Needs to be looked at and verified."
        n284 = disable-structure shown="Enabled" {
          frame Disabled {
            n285 = local write "Status : CapRun"(FALSE ("Status : CapRun")) -> ()
          }
          frame Enabled {
          }
        }
        n286 = control-ref of="Status : CapRun"() -> (w258:refnum<vi>)
        n287 = property class="Bool (strict)"(reference=w258, "Value"=FALSE ("Status : CapRun")) -> ()  [unwired: 1 in, 2 out]
        n288 = call "Message_dialog.vi"("error in (no error)"="Generate Report : error in", "set delay"=2.0, "String"="** Finish Testing **\n\nPreparing Full Report...\n\n" ("message")) -> ("error out"=w254:errorcluster)  [unwired: 8 in]
        n289 = call "Set_K2400_ZeroV.vi"("error in"="Test Finishing : Error in") -> ("error out"=w262:errorcluster)  [unwired: 10 in]
        n290 = call "Set_K2400_Output_Off.vi"("error in (no error)"=w262) -> ("error out"=w261:errorcluster)  [unwired: 10 in]
        n291 = control-ref of="Report Array Header"() -> (w263:refnum<vi>)
        n292 = control-ref of="XY Graph"() -> (w256:refnum<vi>)
        n293 = call "Config_3457_Norm.vi"("error in (no error)"=w261) -> ("error out"=→"Test Finishing : Error Out":errorcluster)  [unwired: 10 in]
        n294 = control-ref of="Temporary test data"() -> (w264:refnum<vi>)
        n295 = call "Ref_Num_Combine_Full_Report.vi"("Temporary test data"=w264, "XY Graph NEW"=w256, "error in (no error)"=w254, "Report Array Header"=w263) -> ("error out"=w250:errorcluster)  [unwired: 7 in]
        n296 = call "Message_dialog.vi"("error in (no error)"=w250, "set delay"=6.0, "String"="** Full Report is Ready  **\n\nCan close this Application by\npressing \"X at the upper right corner of this window.\n" ("message")) -> ("error out"=→"Generate Report : error out":errorcluster)  [unwired: 8 in]
      }
    }
  }
  n297 = disable-structure shown="Enabled" {
    frame Disabled {
      n298 = local read "Stop"() -> (w267:bool)
      n299 = Or(x=w267) -> (x .or. y?=w266:bool)  [unwired: 1 in]
      n300 = local write "After Cap run"(w266) -> ()
    }
    frame Enabled {
    }
  }
